vi "SVL Send Data to Waterfall (2D Array).vi"(0 "waterfall ref":refnum<vi>, 1 "axis labels":T1, 5 "waterfall data":dbl[][](array[numeric]) format="%.2f", 7 "f0 and delta f [Hz]":cluster{"f0":dbl, "delta f":dbl} {"delta f" format="%.2f"; "f0" format="%.2f"}, 9 "y0 and delta y":cluster{"y0":dbl, "delta y":dbl}={"y0"=0.0, "delta y"=1.0} {"delta y" format="%.2f"; "y0" format="%.2f"}, 11 "error in (no error)":errorcluster, 12 "settings":T2={"clear graph before redrawing (F)"=FALSE, "set baseline (F)"=FALSE, "baseline"=0.0, "autoscale (T)"=TRUE} {"baseline" format="%.2f"}, 13 "frontmost (T)":bool=TRUE) -> (4 "dup waterfall ref":refnum<vi>, 15 "error out":errorcluster)   [LabVIEW 2017]
doc: "Sends the waterfall data to the waterfall display. You can use this polymorphic VI to send waterfall data to the waterfall display using a 2D array or a cluster. The data type you wire to the <B>waterfall data</B> input determines the polymorphic instance to use."
uses:
  <vilib>/addons/Sound and Vibration/compatibility/Waterfall/subVIs/svl_Waterfall Global.vi
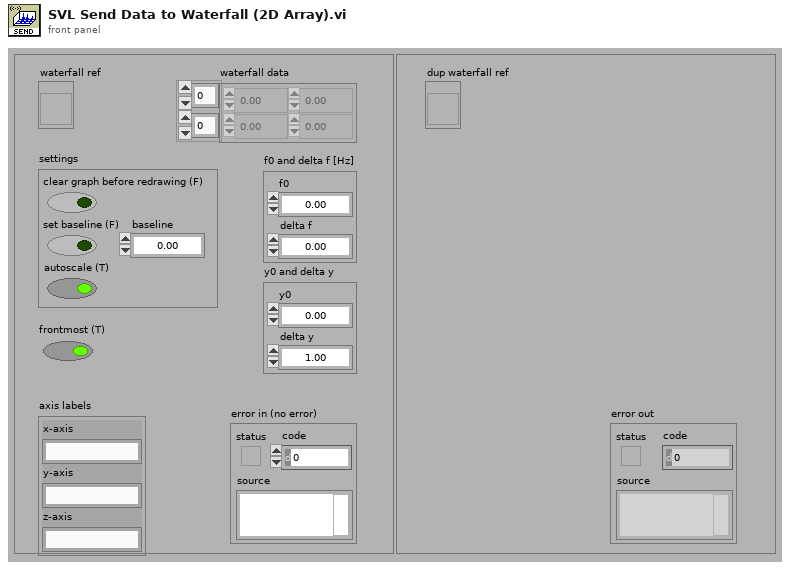
[diagram p1: front panel]
types:
  T1 = cluster{"x-axis":string, "y-axis":string, "z-axis":string}
  T2 = cluster{"clear graph before redrawing (F)":bool, "set baseline (F)":bool, "baseline":dbl, "autoscale (T)":bool}
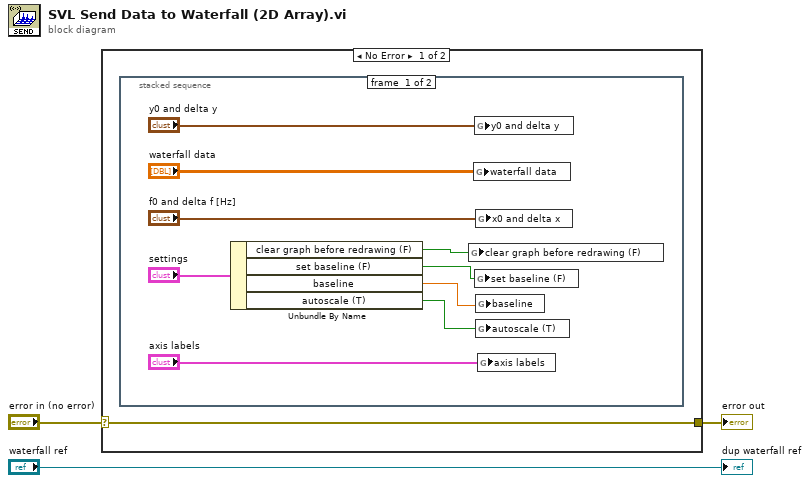
[diagram p0: block diagram]
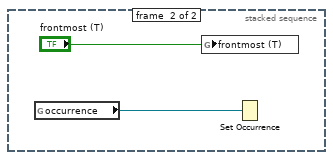
[diagram p2: hidden frame]
diagram:
  n1 = case shown="No Error" "error in (no error)" {
    selector: "error in (no error)" -> [w4 w16]
    tunnel: [w4 w16] -> w1
    frame No Error {
      n2 = stacked-sequence {
        frame #0 {
          n3 = Unbundle By Name("settings") -> ("clear graph before redrawing (F)"=w11:bool, "set baseline (F)"=w10:bool, "baseline"=w9:dbl, "autoscale (T)"=w8:bool)
          n4 = global write "svl_Waterfall Global.vi" "clear graph before redrawing (F)"(w11) -> ()
          n5 = global write "svl_Waterfall Global.vi" "waterfall data"("waterfall data") -> ()
          n6 = global write "svl_Waterfall Global.vi" "y0 and delta y"("y0 and delta y") -> ()
          n7 = global write "svl_Waterfall Global.vi" "set baseline (F)"(w10) -> ()
          n8 = global write "svl_Waterfall Global.vi" "x0 and delta x"("f0 and delta f [Hz]") -> ()
          n9 = global write "svl_Waterfall Global.vi" "baseline"(w9) -> ()
          n10 = global write "svl_Waterfall Global.vi" "autoscale (T)"(w8) -> ()
          n11 = global write "svl_Waterfall Global.vi" "axis labels"("axis labels") -> ()
        }
        frame #1 {
          n12 = global read "svl_Waterfall Global.vi" "occurrence"() -> (w14:refnum<k4>)
          n13 = global write "svl_Waterfall Global.vi" "frontmost (T)"("frontmost (T)") -> ()
          n14 = Set Occurrence(w14) -> ()
        }
      }
    }
    frame Error {
    }
  }
  "error out" <- w1
  "dup waterfall ref" <- "waterfall ref"
